vi "PCO_SetDateTime.vi"(0 "ph":u64, 5 "lvTimestamp":timestamp, 11 "error in (no error)":errorcluster {"code" format="%x"}) -> (4 "ph out":u64, 6 "ErrorMessage":i32 format="%x", 15 "error out":errorcluster {"code" format="%x"})   [LabVIEW 2019, in "SDK.lvlib" / "RecordingControl.lvlib"]
doc: "<b>Description:</b>\nThis function does set date and time information for the internal camera clock, which is used for the timestamp function. When powering up the camera the camera clock is reset and all date and time information is set to zero. If timestamp data should be synchronized with the PC time, this function must be called at least once. It might be necessary to call the function again in distinct time intervals, because some deviation between PC time and camera time might occur after some time. When this function is called the [ms] and [ìs] values of the camera clock are set to zero. All parameter values must be set in packed BCD code.\nThe PCO_SetDateTime function is called during a PCO_OpenCamera call to synchronize PC time with camera time.\n\n<b>Supported camera type:</b>\nAll cameras\n\n<b>Descriptor dependency:</b>\nNone"
uses:
  RecordingControl.lvlib
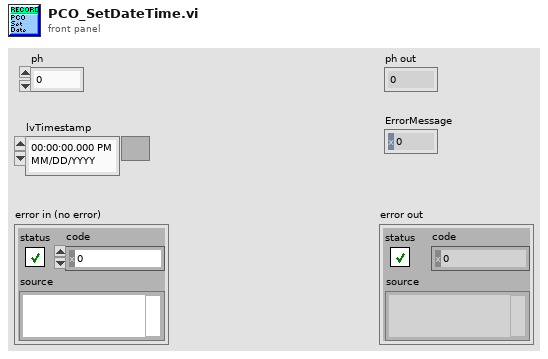
[diagram p1: front panel]
types:
  T1 = typedef "LVDateTimeRec.ctl" = cluster{"fractional second":dbl, "second":i32, "minute":i32, "hour":i32, "day of month":i32, "month":i32, "year":i32, "day of week":i32, "day of year":i32, "DST":i32}
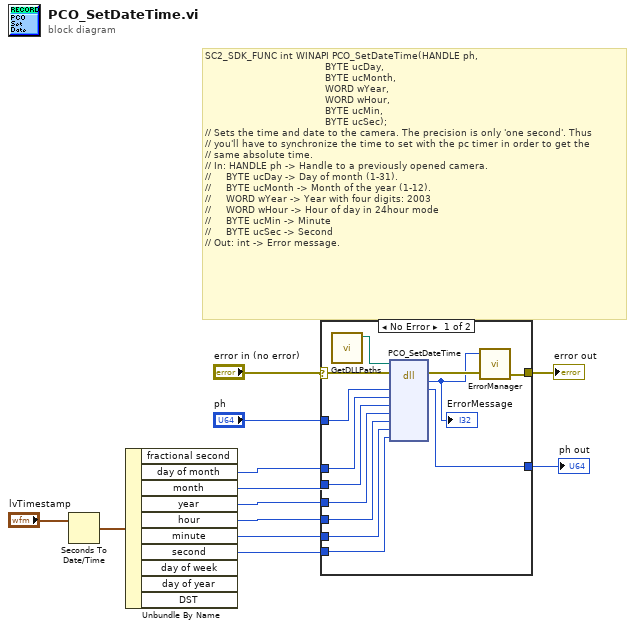
[diagram p0: block diagram]
diagram:
  # "SC2_SDK_FUNC int WINAPI PCO_SetDateTime(HANDLE ph,\n                                        BYTE ucDay,\n                                        BYTE ucMonth,\n                                        WORD wYear,\n                                        WORD wHour,\n                                        BYTE ucMin,\n                                        BYTE ucSec);\n// Sets the time and date to the camera. The precision is only 'one second'. Thus\n// you'll have to synchronize the time to set with the pc timer in order to get the\n// same absolute time.\n// In: HANDLE ph -> Handle to a previously opened camera.\n//     BYTE ucDay -> Day of month (1-31).\n//     BYTE ucMonth -> Month of the year (1-12).\n//     WORD wYear -> Year with four digits: 2003\n//     WORD wHour -> Hour of day in 24hour mode\n//     BYTE ucMin -> Minute\n//     BYTE ucSec -> Second\n// Out: int -> Error message."
  n1 = Seconds To Date/Time(time stamp (now)="lvTimestamp") -> (date time rec=w7:T1)  [unwired: 1 in]
  n2 = Unbundle By Name(w7) -> ("day of month"=w6:i32, "month"=w5:i32, "year"=w4:i32, "hour"=w3:i32, "minute"=w2:i32, "second"=w1:i32)  [unwired: 4 out]
  n3 = case shown="No Error" "error in (no error)" {
    selector: "error in (no error)" -> [w17 w27]
    tunnel: "ph" -> [w25 w26]
    tunnel: [w24 w26] -> w11
    tunnel: w6 -> [w23 _]
    tunnel: w5 -> [w22 _]
    tunnel: w4 -> [w21 _]
    tunnel: w3 -> [w20 _]
    tunnel: w2 -> [w19 _]
    tunnel: w1 -> [w18 _]
    tunnel: [w15 w27] -> w10
    frame No Error {
      n4 = call "GetDLLPaths.vi"() -> ("SC2_Cam_Path"=w13:path)  [unwired: 8 in, 3 out]
      n5 = dll-call lib="?" fn="PCO_SetDateTime"(path in=w13, error in=w17, "ph"=w25, "ucDay"=w23, "ucMonth"=w22, "wYear"=w21, "wHour"=w20, "ucMin"=w19, "ucSec"=w18) -> (error out=w16:errorcluster, "return type"=w14:i32, "ph"=w24:u64)  [unwired: 7 in, 1 out]
      "ErrorMessage" <- w14
      n6 = call "ErrorManager.vi"("error in (no error)"=w16, "error code"=w14) -> ("error out"=w15:errorcluster)  [unwired: 2 in, 1 out]
    }
    frame Error {
    }
  }
  "ph out" <- w11
  "error out" <- w10
